vi "Main.vi"(11 "Module Admin":refnum<class "Delacor_lib_QMH_Cloneable Module Admin.lvclass">) -> ()   [LabVIEW 2024, in "Mensajes.lvlib"]
doc: "This template is based off of the Queued Message Handler design pattern and the Queued Message Handler project template that ships with LabVIEW.\n\nThe main difference is that the queue is private to this module and communication between modules is performed via Broadcast and Request events.\n\nRequest events are wrapped in public API methods and are handled in the Event Handling Loop (EHL) of this VI. Any module can register for Broadcast events sent by this module. The EHL generates messages based on user interface actions.\n\nThe Message Handling Loop (MHL) processes messages generated by the EHL, or by other messages. The messages are string values, so new messages can be added easily to the Message Cases case structure in the MHL. Each message cluster can also provide an optional value for Message Data, which is a variant that can be converted to whatever message-specific data is required.\n_____\nBased on DQMH Dev Tools: Project Template 7.1.0.1503."
uses:
  Mensajes.lvlib
  <vilib>/Delacor/Delacor QMH/Libraries/Cloneable Module Admin_class/Delacor_lib_QMH_Cloneable Module Admin.lvclass/Delacor_lib_QMH_Cloneable Module Admin.ctl
  <vilib>/Delacor/Delacor QMH/Libraries/Message Queue_class/Delacor_lib_QMH_Message Queue.lvclass/Delacor_lib_QMH_Message Queue.ctl
  <vilib>/Delacor/Delacor QMH/Libraries/Module Admin_class/Delacor_lib_QMH_Module Admin.lvclass/Delacor_lib_QMH_Module Admin.ctl
  <vilib>/Delacor/Delacor QMH/Libraries/Message Queue_class/Delacor_lib_QMH_Message Queue.lvclass
  Module Data--cluster.ctl
  <vilib>/Delacor/Delacor QMH/Libraries/Message Queue_class/Delacor_lib_QMH_Enqueue Message (Single).vi
  Stop Argument--cluster.ctl
  <vilib>/Delacor/Delacor QMH/Libraries/Cloneable Module Admin_class/Delacor_lib_QMH_Cloneable Module Admin.lvclass
  Draw FP in Subpanel Argument--cluster.ctl
  Remove From Subpanel Argument--cluster.ctl
  Despliega Mensaje Argument--cluster.ctl
  <vilib>/Utility/miscctls.llb/LVFontTypeDef.ctl
  Set Text Font Settings Argument--cluster.ctl
panel:
  out "Msg":string
  out "error out":errorcluster
  out "Status":string
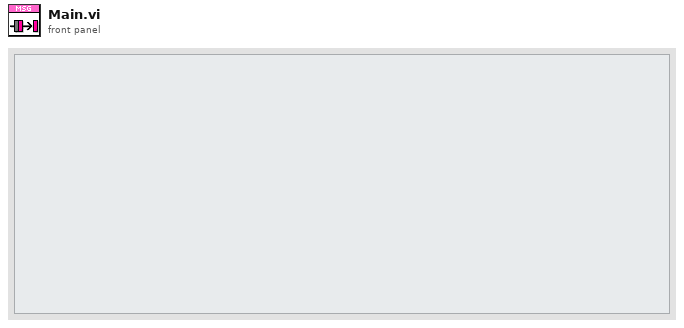
[diagram p1: front panel]
types:
  T1 = typedef "Mensajes.lvlib/Request Events--cluster.ctl" = cluster{"Stop Module":refnum<user-event>, "Show Panel":refnum<user-event>, "Hide Panel":refnum<user-event>, "Show Diagram":refnum<user-event>, "Get Module Execution Status":refnum<user-event>, "Draw FP in Subpanel":refnum<user-event>, "Remove From Subpanel":refnum<user-event>, "Despliega Mensaje":refnum<user-event>, "Set Text Font Settings":refnum<user-event>}
  T2 = typedef "Mensajes.lvlib/Module Data--cluster.ctl" = cluster{"Status":string, "Sub Panel":refnum<vi>, "Msg Ref":refnum<vi>}
  T3 = enum32{"invalid lock state", "Not Locked", "Locked (No Password)", "Password-protected"}
  T4 = typedef "Mensajes.lvlib/Stop Argument--cluster.ctl" = cluster{"Module ID":i32, "Origin":string, "Exit via Stop Module Req?":bool, "Wait for Module to stop?":bool}
  T5 = typedef "Mensajes.lvlib/Draw FP in Subpanel Argument--cluster.ctl" = cluster{"Module ID":i32, "Sub Panel":refnum<vi>}
  T6 = typedef "Mensajes.lvlib/Remove From Subpanel Argument--cluster.ctl" = cluster{"Module ID":i32, "Boolean":bool}
  T7 = typedef "Mensajes.lvlib/Despliega Mensaje Argument--cluster.ctl" = cluster{"Module ID":i32, "Mensaje":string}
  T8 = typedef "Mensajes.lvlib/Set Text Font Settings Argument--cluster.ctl" = cluster{"Module ID":i32, "Text.Font":T9}
  T9 = typedef "LVFontTypeDef.ctl" = cluster{"Font Name":string, "Size":u16, "Bold":bool, "Italic":bool, "Underline":bool, "Strikeout":bool, "Color":u32}
  T10 = enum32{"Invalid", "Standard", "Closed", "Hidden", "Minimized", "Maximized"}
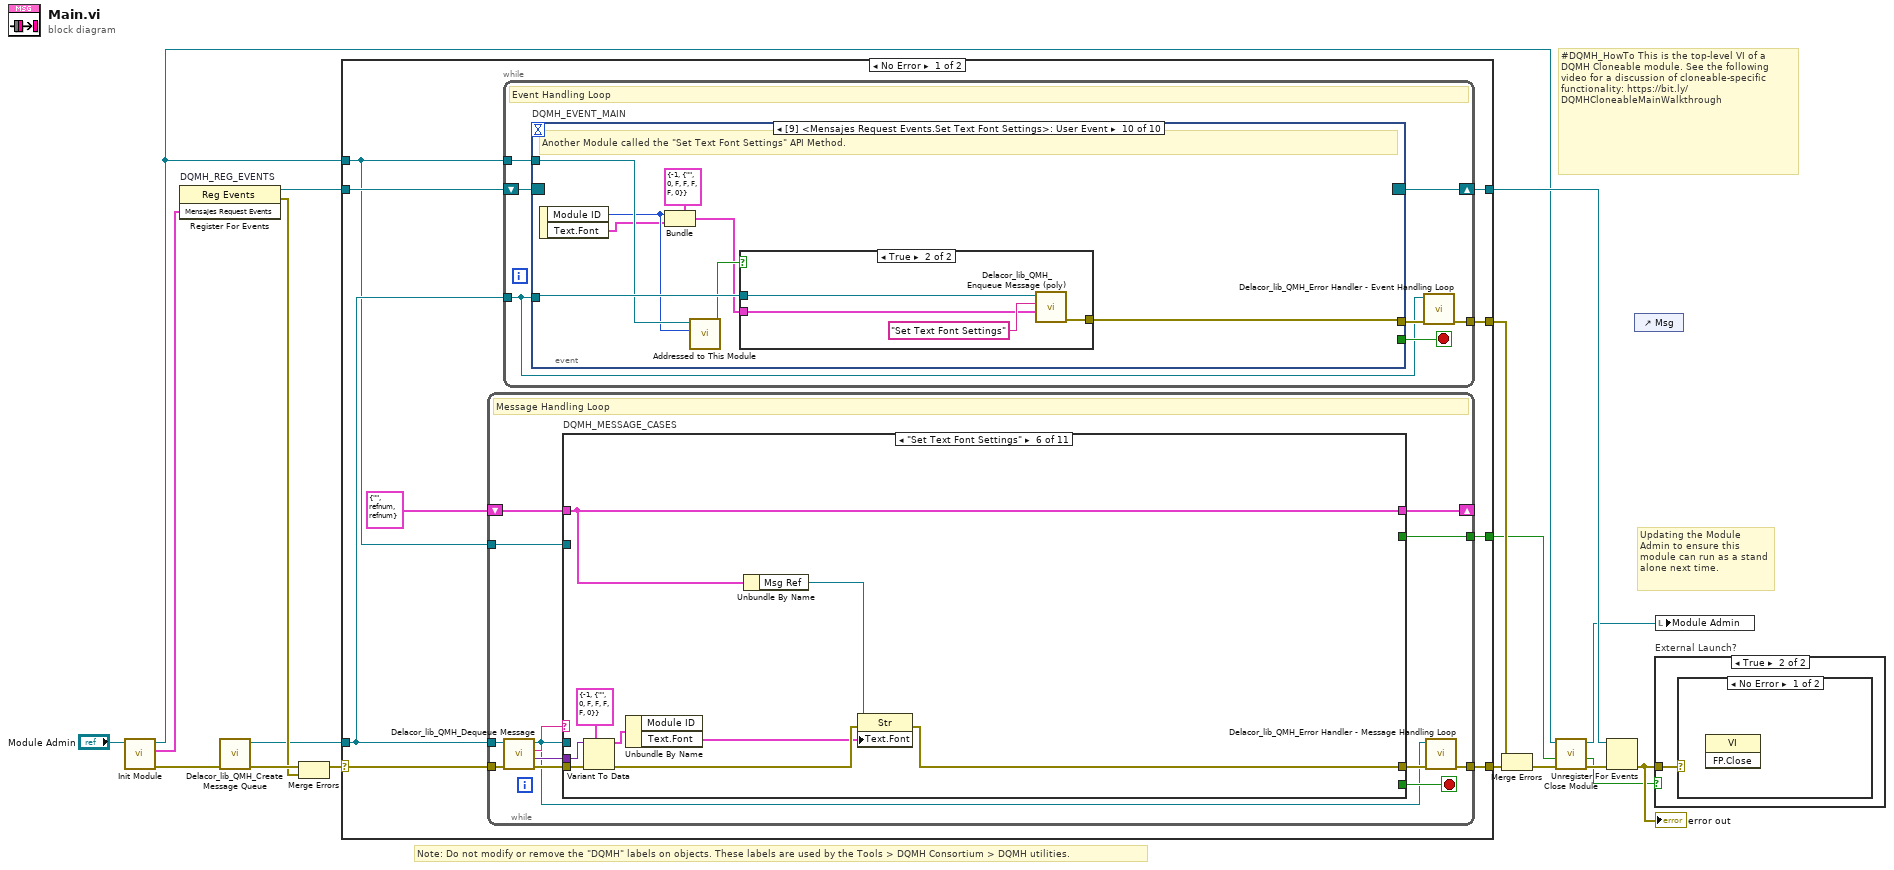
[diagram p0: block diagram]
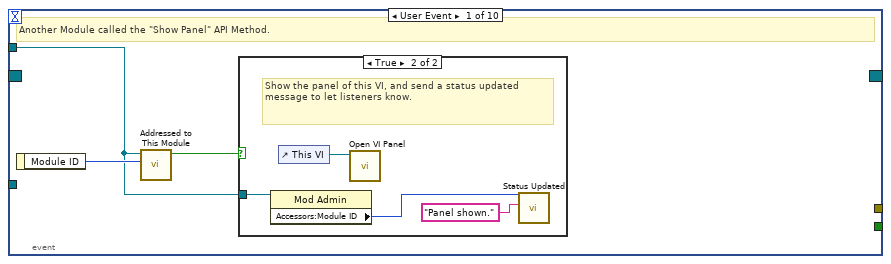
[diagram p2: hidden frame]
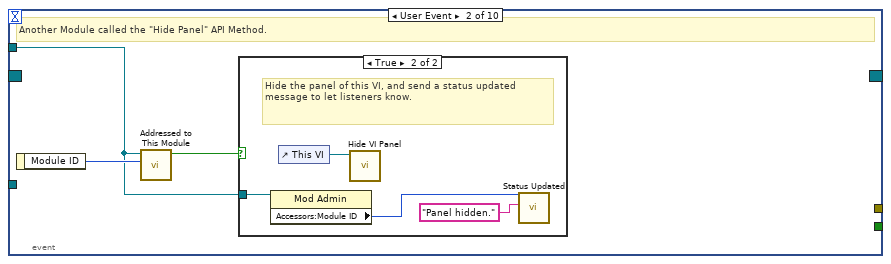
[diagram p4: hidden frame]
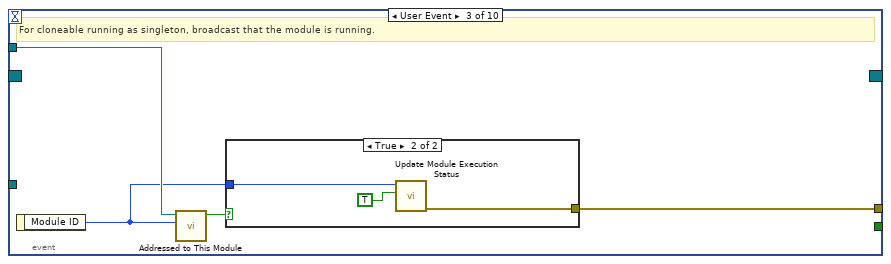
[diagram p6: hidden frame]
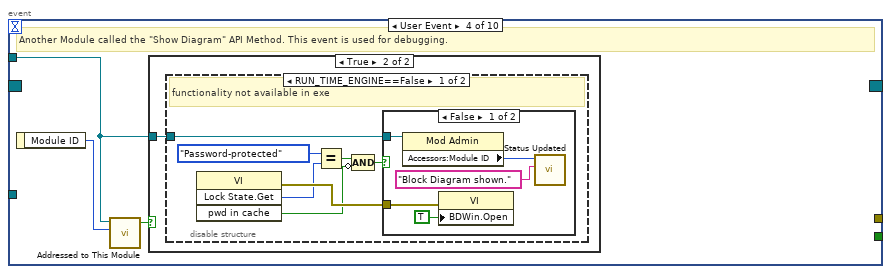
[diagram p8: hidden frame]
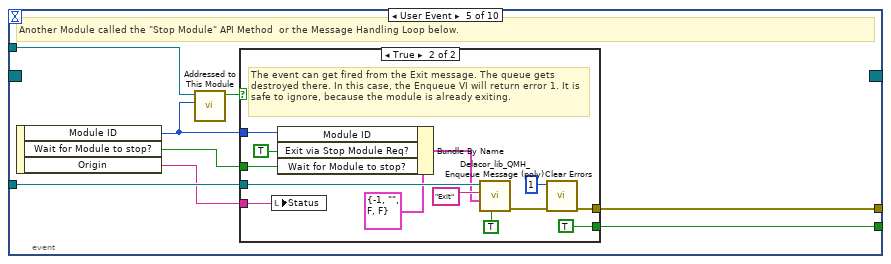
[diagram p12: hidden frame]
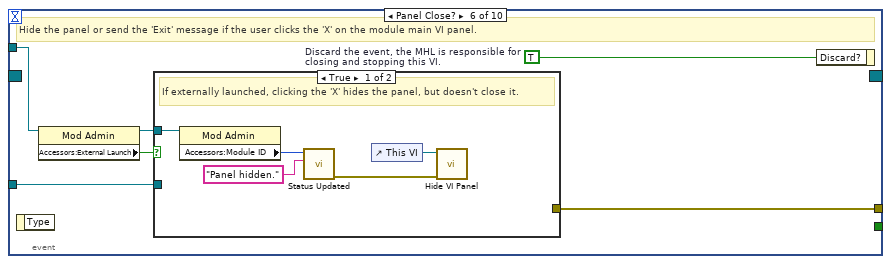
[diagram p14: hidden frame]
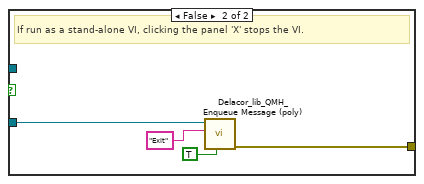
[diagram p15: hidden frame]
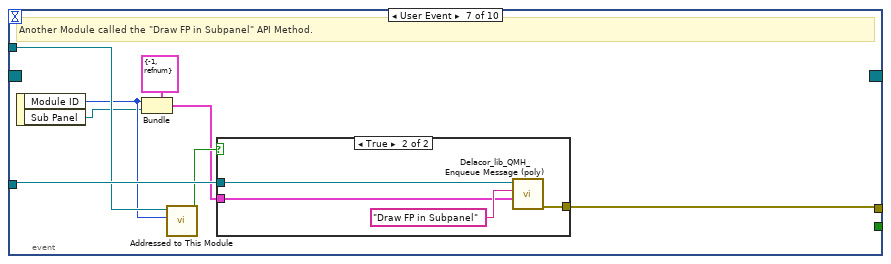
[diagram p16: hidden frame]
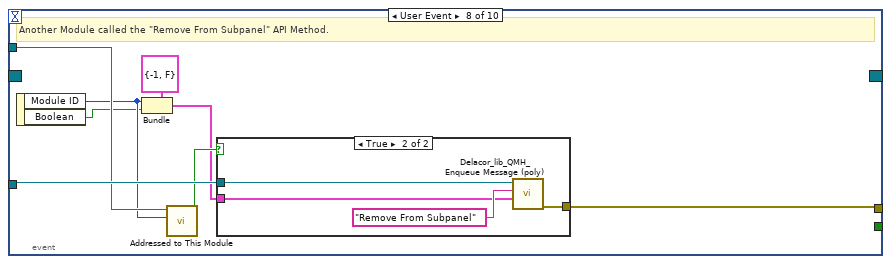
[diagram p18: hidden frame]
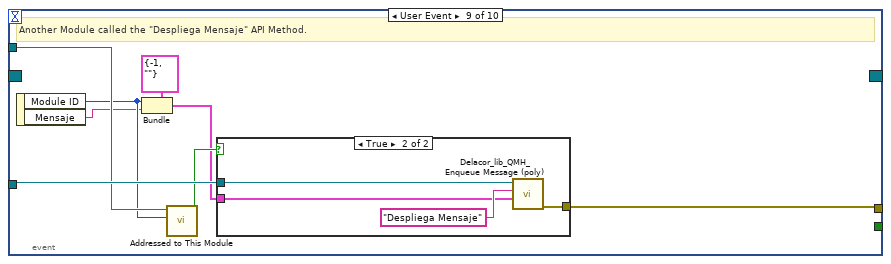
[diagram p20: hidden frame]
diagram:
  # "#DQMH_HowTo This is the top-level VI of a DQMH Cloneable module. See the following video for a discussion of cloneable-specific functionality: https://bit.ly/DQMHCloneableMainWalkthrough"
  # "Note: Do not modify or remove the \"DQMH\" labels on objects. These labels are used by the Tools > DQMH Consortium > DQMH utilities."
  # "Updating the Module Admin to ensure this module can run as a stand alone next time."
  n1 = call "Init Module.vi"("Cloneable Module Admin in"="Module Admin") -> ("error out"=w15:errorcluster, "Mensajes Request Events"=w7:T1, "Cloneable Module Admin out"=w4:refnum<class "Delacor_lib_QMH_Cloneable Module Admin.lvclass">)  [unwired: 8 in]
  n2 = register-events "DQMH_REG_EVENTS"(w7) -> (reference out=w8:refnum<event-registration>, error out=w10:errorcluster)  [unwired: 2 in]
  n3 = call <vilib>:"Delacor_lib_QMH_Create Message Queue.vi"("error in"=w15) -> ("error out"=w12:errorcluster, "Message Queue"=w6:refnum<class "Delacor_lib_QMH_Message Queue.lvclass">)  [unwired: 9 in]
  n4 = Merge Errors(w12, w10) -> (w11:errorcluster)
  n5 = case shown="No Error" w11 {
    selector: w11 -> [w25 w317]
    tunnel: [w27 w316] -> w16
    tunnel: [w24 w315] -> w9
    tunnel: w8 -> [w22 w315]
    tunnel: w6 -> [w21 w308]
    tunnel: [w26 _] -> w17
    tunnel: w4 -> [w20 w311]
    tunnel: [w19 _] -> w2
    frame No Error {
      n6 = while {
        tunnel: w21 -> [w156]
        shift-right: [w163] -> _
        shift-left: T2 {"Status"="", "Sub Panel"=refnum, "Msg Ref"=refnum} ("Data Cluster") -> [w164]
        tunnel: w25 -> [w167]
        tunnel: [w165] -> w27
        tunnel: w20 -> [w158]
        tunnel: [w157] -> w19
        stop <- w162 stop-if-true
        # "Message Handling Loop"
        n7 = call-dynamic "Delacor_lib_QMH_Dequeue Message.vi"("error in"=w167, "Message Queue in"=w156) -> ("error out"=w166:errorcluster, "Message Data"=w160:variant, "Message"=w161:string, "Message Queue out"=w159:refnum<class "Delacor_lib_QMH_Message Queue.lvclass">)  [unwired: 6 in]
        n8 = case "DQMH_MESSAGE_CASES" shown="\"Set Text Font Settings\"" w161 {
          selector: w161 -> [_ _ _ _ _ _ _ _ _ _ w297]
          tunnel: w159 -> [_ _ _ _ _ _ _ _ w261 w289 _]
          tunnel: w166 -> [w187 w191 w210 w230 w245 w254 w257 w259 w271 w295 w306]
          tunnel: [w185 w191 w206 w228 w243 w249 w256 w259 w267 w290 w307] -> w168
          tunnel: w164 -> [w178 w190 w196 w222 w244 w247 w255 w258 w265 w279 w304]
          tunnel: [w177 w190 w197 w218 w244 w247 w255 w258 w265 w279 w304] -> w163
          tunnel: [_ _ _ _ _ _ _ _ _ w288 _] -> w162
          tunnel: w160 -> [_ _ w205 w227 w242 w253 _ _ w264 w286 _]
          tunnel: w158 -> [w173 _ w194 w221 w238 _ _ _ w263 w281 w303]
          tunnel: [_ _ _ _ _ _ _ _ _ w284 _] -> w157
          frame "Initialize" {
            w171 = "Initial Message" ("Initial Message")
            # "#DQMH_CodeNeeded - Initialize the appearance of the front panel."
            # "Initialize - Any operation that needs to be done before the module can receive messages. Synchronize Caller Events.vi will inform Start Module.vi that the module has launched and is ready to receive messages. Module Did Init.vi will broadcast that the module initialized."
            n9 = call "Synchronize Caller Events.vi"("error in"=w187, "Module Admin"=w173) -> ("error out"=w186:errorcluster, "Module Admin out"=w172:refnum<class "Delacor_lib_QMH_Cloneable Module Admin.lvclass">)  [unwired: 8 in]
            n10 = property on="Property Node" class="Mod Admin"(reference=w172) -> ("Accessors:Module ID"=w170:i32, "Accessors:External Launch"=w174:bool)  [unwired: 1 in, 2 out]
            n11 = call "Module Name--constant.vi"("Module ID"=w170) -> ("Module Name"=w182:string)  [unwired: 10 in]
            n12 = property on="Property Node" class="VI"("Front Panel.Title"=w182) -> (reference out=w184:refnum<vi>, error out=w189:errorcluster)  [unwired: 2 in]
            n13 = Select(t=T10."Hidden" ("State"), s=w174, f=T10."Standard" ("State")) -> (s? t:f=w179:T10)
            n14 = control-ref of="Msg"() -> (w169:refnum<vi>)
            n15 = invoke on="Invoke Node" class="VI" method="FP.Open"(reference=w184, error in=w189, "State"=w179) -> (reference out=w183:refnum<vi>, error out=w188:errorcluster)  [unwired: 2 in, 3 out]
            n16 = Bundle By Name(cluster=w178, "Msg Ref"=w169, "Status"=w171) -> (w177:T2)
            n17 = invoke on="Invoke Node" class="VI" method="FP.Center"(reference=w183, error in=w188) -> ()  [unwired: 1 in, 3 out]
            n18 = call "Module Name--constant.vi"("Module ID"=w170) -> ("Module Name"=w175:string)  [unwired: 10 in]
            n19 = call "Module Did Init.vi"("error in"=w186, "Initialized?"=TRUE, "Origin"=w175, "Module ID"=w170) -> ("error out"=w185:errorcluster)  [unwired: 7 in]
            "Status" <- w171
          }
          frame "---Module Specific---" {
            # "Separator -- The following cases handle messages specific to this Module."
          }
          frame "Draw FP in Subpanel" {
            # "Draw FP in Subpanel"
            n20 = Variant To Data(error in=w210, type=T5 {"Module ID"=-1, "Sub Panel"=refnum} ("Draw FP in Subpanel Argument"), Variant=w205) -> (data=w203:T5, error out=w207:errorcluster)
            n21 = property class="Mod Admin"(reference=w194) -> ("Accessors:Module ID"=w193:i32)  [unwired: 1 in, 2 out]
            n22 = Unbundle By Name(w203) -> ("Sub Panel"=w195:refnum<vi>)
            n23 = control-ref of="This VI"() -> (w200:refnum<vi>)
            n24 = property class="VI"(reference=w200, error in=w207) -> (reference out=w199:refnum<vi>, error out=w208:errorcluster, "FP.State"=w198:T10)
            n25 = case shown="\"Closed\"" w198 {
              tunnel: [w211 w214] -> w201
              tunnel: [w212 w216] -> w209
              tunnel: w208 -> [w212 w215]
              tunnel: w199 -> [w211 w213]
              frame "Closed" {
              }
              frame "Standard", Default {
                n26 = invoke class="VI" method="FP.Close"(reference=w213, error in=w215) -> (reference out=w214:refnum<vi>, error out=w216:errorcluster)  [unwired: 1 in, 1 out]
              }
            }
            n27 = invoke class="SubPnl" method="Insert VI"(reference=w195, error in=w209, "VI Ref"=w201) -> (reference out=w202:refnum<vi>, error out=w206:errorcluster)  [unwired: 1 in, 2 out]
            n28 = call "Status Updated.vi"("error in"=w206, "Status"="Front Panel Inserted in Subpanel", "Module ID"=w193) -> ()  [unwired: 8 in, 1 out]
            n29 = Bundle By Name(cluster=w196, "Sub Panel"=w202) -> (w197:T2)
          }
          frame "Remove From Subpanel" {
            # "Remove From Subpanel"
            n30 = Variant To Data(error in=w230, type=T6 {"Module ID"=-1, "Boolean"=FALSE} ("Remove From Subpanel Argument"), Variant=w227) -> (data=w225:T6, error out=w229:errorcluster)
            n31 = Unbundle By Name(w225) -> ()  [unwired: 2 out]
            n32 = property class="Mod Admin"(reference=w221) -> ("Accessors:Module ID"=w220:i32)  [unwired: 1 in, 2 out]
            n33 = Unbundle By Name(w222) -> ("Sub Panel"=w224:refnum<vi>)
            n34 = Not A Number/Path/Refnum?(number/path/refnum=w224) -> (NaN/Path/Refnum?=w223:bool)
            n35 = case shown="False" w223 {
              tunnel: w229 -> [w234 w236]
              tunnel: [w233 w236] -> w228
              tunnel: w224 -> [w232 _]
              tunnel: ["Panel Removed from Subpanel" "This module has not been inserted into the subpanel"] -> w219
              frame False {
                n36 = invoke class="SubPnl" method="Remove VI"(reference=w232, error in=w234) -> (error out=w233:errorcluster)  [unwired: 1 in, 2 out]
              }
              frame True {
              }
            }
            n37 = Bundle By Name(cluster=w222, "Sub Panel"=refnum<vi> refnum) -> (w218:T2)
            n38 = call "Status Updated.vi"("error in"=w228, "Status"=w219, "Module ID"=w220) -> ()  [unwired: 8 in, 1 out]
          }
          frame "Despliega Mensaje" {
            n39 = Variant To Data(error in=w245, type=T7 {"Module ID"=-1, "Mensaje"=""} ("Despliega Mensaje Argument"), Variant=w242) -> (data=w240:T7, error out=w243:errorcluster)
            n40 = property class="Mod Admin"(reference=w238) -> ("Accessors:Module ID"=w237:i32)  [unwired: 1 in, 2 out]
            n41 = Unbundle By Name(w240) -> ("Mensaje"=w239:string)  [unwired: 1 out]
            "Msg" <- w239
            n42 = call "Status Updated.vi"("Status"=w239, "Module ID"=w237) -> ()  [unwired: 9 in, 1 out]
          }
          frame "Set Text Font Settings" {
            n43 = Variant To Data(error in=w254, type=T8 {"Module ID"=-1, "Text.Font"={"Font Name"="", "Size"=0, "Bold"=FALSE, "Italic"=FALSE, "Underline"=FALSE, "Strikeout"=FALSE, "Color"=0}} ("Set Text Font Settings Argument"), Variant=w253) -> (data=w251:T8, error out=w250:errorcluster)
            n44 = Unbundle By Name(w251) -> ("Text.Font"=w248:T9)  [unwired: 1 out]
            n45 = Unbundle By Name(w247) -> ("Msg Ref"=w246:refnum<vi>)
            n46 = property class="Str"(reference=w246, error in=w250, "Text.Font"=w248) -> (error out=w249:errorcluster)  [unwired: 1 out]
          }
          frame "---Copy This Frame---" {
            # "Duplicate this frame when creating new messages.  Change this comment in the duplicated frame to describe this message."
            n47 = Merge Errors(w257) -> (w256:errorcluster)
          }
          frame "---Exit and Error Handling---" {
            # "Separator - the following cases handle errors and exit messages."
          }
          frame "Error" {
            # "#DQMH_CodeRecommended - If the module is running in standalone mode (External Launch = FALSE), this code will pop up an error dialog and call the 'Exit' message if an error occurs. Add more fine-grained error management here."
            # "Error - Check the error message data and respond accordingly. This message is sent by the \"Error Handler\" VIs at the end of each loop in this application."
            n48 = property on="Property Node" class="Mod Admin"(reference=w263) -> ("Accessors:External Launch"=w262:bool, "Accessors:Module ID"=w260:i32)  [unwired: 1 in, 2 out]
            n49 = Variant To Data(error in=w271, type=errorcluster {"status"=FALSE, "code"=0, "source"=""} ("error constant"), Variant=w264) -> (data=w266:errorcluster, error out=w269:errorcluster)
            n50 = local write "error out"(w266) -> ()
            n51 = call "Error Reported.vi"("Error"=w266, "Module ID"=w260) -> ()  [unwired: 9 in, 1 out]
            n52 = case shown="False" w262 {
              tunnel: [w276 _] -> w268
              tunnel: w261 -> [w274 _]
              tunnel: w266 -> [w275 _]
              frame False {
                n53 = disable-structure shown="Default" {
                  disable-tunnel: w275 -> [w277 _]
                  frame condition #0 (active) {
                    # "If the module is running standalone, then pop up an error dialog and call the \"Exit\" message."
                    n54 = call <vilib>:"Simple Error Handler.vi"("error in (no error)"=w277) -> ()  [unwired: 4 in, 5 out]
                  }
                  frame condition #1 {
                    # "To prevent the Simple Error Handler VI from being loaded (e.g. when deploying to a Real-Time target), add the Conditional Disable Symbol \"DQMH_Disable_SEH\" to your project and set it to TRUE."
                  }
                }
                n55 = call-poly <vilib>:"Delacor_lib_QMH_Enqueue Message (poly).vi"("Priority Message? (F)"=TRUE, "Message"="Exit", "Message Queue in"=w274) -> ("error out"=w276:errorcluster)  [unwired: 7 in, 1 out]
              }
              frame True {
                # "If the module was launched externally, calling the Error Reported broadcast VI is the only action performed by the \"Error\" message. The module's caller can then process the error appropriately."
              }
            }
            n56 = Merge Errors(w269, w268) -> (w267:errorcluster)
          }
          frame "Exit" {
            w287 = 91  # 91: not all Exit messages will have an argument
            w288 = TRUE  # Stop the VI
            # "Release the message queue reference"
            # "#DQMH_CodeNeeded - Add any required cleanup code here."
            # "Exit - Exit the application."
            n57 = Variant To Data(error in=w295, type=T4 {"Module ID"=-1, "Origin"="", "Exit via Stop Module Req?"=FALSE, "Wait for Module to stop?"=FALSE} ("Stop Argument"), Variant=w286) -> (data=w283:T4, error out=w291:errorcluster)
            n58 = call <vilib>:"Clear Errors.vi"("error in (no error)"=w291, "specific error code to clear (0: all)"=w287) -> ("error out"=w294:errorcluster)  [unwired: 4 in, 1 out]
            n59 = property on="Property Node" class="Mod Admin"(reference=w281) -> ("Accessors:Module ID"=w280:i32)  [unwired: 1 in, 2 out]
            n60 = control-ref of="This VI"() -> (w282:refnum<vi>)
            n61 = call-dynamic "Delacor_lib_QMH_Release Message Queue.vi"("error in"=w294, "Message Queue"=w289) -> ("error out"=w293:errorcluster)  [unwired: 9 in]
            n62 = call "Handle Exit.vi"("Stop Argument"=w283, "Module Admin in"=w281, "VI reference"=w282) -> ("error out"=w292:errorcluster, "Wait for Stop?"=w284:bool)  [unwired: 7 in]
            n63 = Merge Errors(w293, w292) -> (w290:errorcluster)
            n64 = Unbundle By Name(w279) -> ("Sub Panel"=w278:refnum<vi>)
            n65 = call "Error Reported.vi"("Error"=w290, "Module ID"=w280) -> ()  [unwired: 9 in, 1 out]
            n66 = invoke class="SubPnl" method="Remove VI"(reference=w278) -> ()  [unwired: 2 in, 3 out]
          }
          frame Default {
            # "'Default' case only runs if there is a message that isn't defined in any of the other cases.  Output a programming error."
            n67 = property on="Property Node" class="Mod Admin"(reference=w303) -> ("Accessors:Module ID"=w302:i32)  [unwired: 1 in, 2 out]
            n68 = call "Module Name--constant.vi"("Module ID"=w302) -> ("Module Name"=w296:string)  [unwired: 10 in]
            n69 = Format Into String(format string="The invalid message string \"%s\" was received in the Message Handling Loop for module \"%s\".", w297, w296) -> (resulting string=w299:string)  [unwired: 2 in, 1 out]
            n70 = call <vilib>:"Error Cluster From Error Code.vi"("show call chain? (False)"=TRUE, "error message (\"\")"=w299, "error code (0)"=1) -> ("error out"=w305:errorcluster)  [unwired: 6 in]
            n71 = Merge Errors(w306, w305) -> (w307:errorcluster)
          }
        }
        n72 = call-dynamic "Delacor_lib_QMH_Error Handler - Message Handling Loop.vi"("error in"=w168, "Message Queue in"=w159) -> ("dup error in"=w165:errorcluster)  [unwired: 8 in, 1 out]
      }
      n73 = while {
        tunnel: w21 -> [w28]
        shift-right: [w31] -> w24
        shift-left: w22 -> [w32]
        tunnel: [w33] -> w26
        tunnel: w20 -> [w29]
        stop <- w30 stop-if-true
        # "Event Handling Loop"
        n74 = event "DQMH_EVENT_MAIN" shown="[9] <Mensajes Request Events.Set Text Font Settings>: User Event" {
          selector: w32 -> [_ _ _ _ _ _ _ _ _ _]
          dyn-events: [_ _ _ _ _ _ _ _ _ _] -> w31
          timeout: _ -> [_ _ _ _ _ _ _ _ _ _]
          tunnel: [_ _ _ _ w75 _ _ _ _ _] -> w30
          tunnel: w28 -> [_ _ _ _ w78 w95 w114 w126 w139 w151]
          tunnel: [_ _ w52 _ w79 w98 w115 w127 w132 w144] -> w34
          tunnel: w29 -> [w35 w42 w50 w56 w77 w96 w112 w124 w137 w149]
          event User Event {
            # "Another Module called the \"Show Panel\" API Method."
            n75 = event-data() -> ("Module ID"=w36:i32)  [unwired: 1 in]
            n76 = call "Addressed to This Module.vi"("Module ID from Argument"=w36, "Module Admin"=w35) -> ("Addressed to this instance?"=w37:bool)  [unwired: 8 in, 1 out]
            n77 = case shown="True" w37 {
              tunnel: w35 -> [_ w39]
              frame False {
              }
              frame True {
                # "Show the panel of this VI, and send a status updated message to let listeners know."
                n78 = property on="Property Node" class="Mod Admin"(reference=w39) -> ("Accessors:Module ID"=w38:i32)  [unwired: 1 in, 2 out]
                n79 = control-ref of="This VI"() -> (w41:refnum<vi>)
                n80 = call "Open VI Panel.vi"("VI"=w41) -> ()  [unwired: 10 in, 1 out]
                n81 = call "Status Updated.vi"("Status"="Panel shown." ("format string"), "Module ID"=w38) -> ()  [unwired: 9 in, 1 out]
              }
            }
          }
          event User Event {
            # "Another Module called the \"Hide Panel\" API Method."
            n82 = event-data() -> ("Module ID"=w43:i32)  [unwired: 1 in]
            n83 = call "Addressed to This Module.vi"("Module ID from Argument"=w43, "Module Admin"=w42) -> ("Addressed to this instance?"=w44:bool)  [unwired: 8 in, 1 out]
            n84 = case shown="True" w44 {
              tunnel: w42 -> [_ w46]
              frame False {
              }
              frame True {
                # "Hide the panel of this VI, and send a status updated message to let listeners know."
                n85 = property on="Property Node" class="Mod Admin"(reference=w46) -> ("Accessors:Module ID"=w45:i32)  [unwired: 1 in, 2 out]
                n86 = control-ref of="This VI"() -> (w48:refnum<vi>)
                n87 = call "Hide VI Panel.vi"("VI"=w48) -> ()  [unwired: 10 in, 1 out]
                n88 = call "Status Updated.vi"("Status"="Panel hidden." ("format string"), "Module ID"=w45) -> ()  [unwired: 9 in, 1 out]
              }
            }
          }
          event User Event {
            # "For cloneable running as singleton, broadcast that the module is running."
            n89 = event-data() -> ("Module ID"=w49:i32)  [unwired: 1 in]
            n90 = call "Addressed to This Module.vi"("Module ID from Argument"=w49, "Module Admin"=w50) -> ("Addressed to this instance?"=w51:bool)  [unwired: 8 in, 1 out]
            n91 = case shown="True" w51 {
              tunnel: [_ w55] -> w52
              tunnel: w49 -> [_ w54]
              frame False {
              }
              frame True {
                n92 = call "Update Module Execution Status.vi"("Running?"=TRUE, "Module ID"=w54) -> ("error out"=w55:errorcluster)  [unwired: 9 in]
              }
            }
          }
          event User Event {
            # "Another Module called the \"Show Diagram\" API Method. This event is used for debugging."
            n93 = event-data() -> ("Module ID"=w57:i32)  [unwired: 1 in]
            n94 = call "Addressed to This Module.vi"("Module ID from Argument"=w57, "Module Admin"=w56) -> ("Addressed to this instance?"=w58:bool)  [unwired: 8 in, 1 out]
            n95 = case shown="True" w58 {
              tunnel: w56 -> [_ w59]
              frame False {
              }
              frame True {
                n96 = disable-structure shown="RUN_TIME_ENGINE==False" {
                  disable-tunnel: w59 -> [w60 _]
                  frame condition #0 (active) {
                    # "functionality not available in exe"
                    n97 = invoke on="Invoke Node" class="VI" method="Lock State.Get"() -> (error out=w66:errorcluster, "Get Lock State"=w65:T3, "pwd in cache"=w62:bool)  [unwired: 4 in, 1 out]
                    n98 = Equal?(x=T3."Password-protected", y=w65) -> (x = y?=w63:bool)
                    n99 = Compound Arithmetic op=AND(w63, invert w62) -> (w61:bool)
                    n100 = case shown="False" w61 {
                      tunnel: w66 -> [w71 _]
                      tunnel: w60 -> [w68 _]
                      frame False {
                        n101 = property on="Property Node" class="Mod Admin"(reference=w68) -> ("Accessors:Module ID"=w67:i32)  [unwired: 1 in, 2 out]
                        n102 = property on="Property Node" class="VI"(error in=w71, "BDWin.Open"=TRUE ("Block Diagram Window:Open")) -> ()  [unwired: 1 in, 2 out]
                        n103 = call "Status Updated.vi"("Status"="Block Diagram shown." ("format string"), "Module ID"=w67) -> ()  [unwired: 9 in, 1 out]
                      }
                      frame True {
                        # "Password-protected VI, and the password is not in the cache. Do not show the diagram."
                      }
                    }
                  }
                  frame condition #1 {
                  }
                }
              }
            }
          }
          event User Event {
            # "Another Module called the \"Stop Module\" API Method  or the Message Handling Loop below."
            n104 = event-data() -> ("Module ID"=w73:i32, "Wait for Module to stop?"=w74:bool, "Origin"=w72:string)  [unwired: 1 in]
            n105 = call "Addressed to This Module.vi"("Module ID from Argument"=w73, "Module Admin"=w77) -> ("Addressed to this instance?"=w76:bool)  [unwired: 8 in, 1 out]
            n106 = case shown="True" w76 {
              tunnel: [_ w91] -> w79
              tunnel: w78 -> [_ w87]
              tunnel: [_ TRUE] -> w75
              tunnel: w74 -> [_ w82]
              tunnel: w73 -> [_ w84]
              tunnel: w72 -> [_ w80]
              frame False {
              }
              frame True {
                # "The event can get fired from the Exit message. The queue gets destroyed there. In this case, the Enqueue VI will return error 1. It is safe to ignore, because the module is already exiting."
                n107 = local write "Status"(w80) -> ()
                n108 = Bundle By Name(cluster=T4 {"Module ID"=-1, "Origin"="", "Exit via Stop Module Req?"=FALSE, "Wait for Module to stop?"=FALSE} ("Stop Argument"), "Module ID"=w84, "Exit via Stop Module Req?"=TRUE, "Wait for Module to stop?"=w82) -> (w81:T4)
                n109 = call-poly <vilib>:"Delacor_lib_QMH_Enqueue Message (poly).vi"("Priority Message? (F)"=TRUE, "Message Data"=w81, "Message"="Exit", "Message Queue in"=w87) -> ("error out"=w92:errorcluster)  [unwired: 6 in, 1 out]
                n110 = call <vilib>:"Clear Errors.vi"("error in (no error)"=w92, "specific error code to clear (0: all)"=1) -> ("error out"=w91:errorcluster)  [unwired: 4 in, 1 out]
              }
            }
          }
          event Panel Close? {
            w97 = TRUE  # Discard the event, the MHL is responsible for closing and stopping this VI.
            # "Hide the panel or send the 'Exit' message if the user clicks the 'X' on the module main VI panel."
            n111 = event-data() -> ()  [unwired: 1 in, 1 out]
            n112 = property on="Property Node" class="Mod Admin"(reference=w96) -> (reference out=w93:refnum<class "Delacor_lib_QMH_Cloneable Module Admin.lvclass">, "Accessors:External Launch"=w94:bool)  [unwired: 1 in, 1 out]
            n113 = case shown="True" w94 {
              tunnel: w95 -> [_ w106]
              tunnel: [_ w107] -> w98
              tunnel: w93 -> [w100 _]
              frame True {
                # "If externally launched, clicking the 'X' hides the panel, but doesn't close it."
                n114 = property on="Property Node" class="Mod Admin"(reference=w100) -> ("Accessors:Module ID"=w99:i32)  [unwired: 1 in, 2 out]
                n115 = call "Status Updated.vi"("Status"="Panel hidden." ("format string"), "Module ID"=w99) -> ("error out"=w103:errorcluster)  [unwired: 9 in]
                n116 = control-ref of="This VI"() -> (w102:refnum<vi>)
                n117 = call "Hide VI Panel.vi"("error in"=w103, "VI"=w102) -> ()  [unwired: 9 in, 1 out]
              }
              frame False {
                # "If run as a stand-alone VI, clicking the panel 'X' stops the VI."
                n118 = call-poly <vilib>:"Delacor_lib_QMH_Enqueue Message (poly).vi"("Priority Message? (F)"=TRUE, "Message"="Exit", "Message Queue in"=w106) -> ("error out"=w107:errorcluster)  [unwired: 7 in, 1 out]
              }
            }
            n119 = event-data ("Event Filter Node")("Discard?"=w97) -> ()  [unwired: 1 in, 1 out]
          }
          event User Event {
            # "Another Module called the \"Draw FP in Subpanel\" API Method."
            n120 = event-data() -> ("Module ID"=w109:i32, "Sub Panel"=w108:refnum<vi>)  [unwired: 1 in]
            n121 = Bundle(cluster=T5 {"Module ID"=-1, "Sub Panel"=refnum} ("Draw FP in Subpanel Argument"), "Module ID"=w109, "Sub Panel"=w108) -> (w110:T5)
            n122 = call "Addressed to This Module.vi"("Module ID from Argument"=w109, "Module Admin"=w112) -> ("Addressed to this instance?"=w113:bool)  [unwired: 8 in, 1 out]
            n123 = case shown="True" w113 {
              tunnel: w114 -> [_ w118]
              tunnel: w110 -> [_ w116]
              tunnel: [_ w119] -> w115
              frame False {
              }
              frame True {
                n124 = call-poly <vilib>:"Delacor_lib_QMH_Enqueue Message (poly).vi"("Message Data"=w116, "Message"="Draw FP in Subpanel", "Message Queue in"=w118) -> ("error out"=w119:errorcluster)  [unwired: 7 in, 1 out]
              }
            }
          }
          event User Event {
            # "Another Module called the \"Remove From Subpanel\" API Method."
            n125 = event-data() -> ("Module ID"=w121:i32, "Boolean"=w120:bool)  [unwired: 1 in]
            n126 = Bundle(cluster=T6 {"Module ID"=-1, "Boolean"=FALSE} ("Remove From Subpanel Argument"), "Module ID"=w121, "Boolean"=w120) -> (w122:T6)
            n127 = call "Addressed to This Module.vi"("Module ID from Argument"=w121, "Module Admin"=w124) -> ("Addressed to this instance?"=w125:bool)  [unwired: 8 in, 1 out]
            n128 = case shown="True" w125 {
              tunnel: w126 -> [_ w130]
              tunnel: w122 -> [_ w128]
              tunnel: [_ w131] -> w127
              frame False {
              }
              frame True {
                n129 = call-poly <vilib>:"Delacor_lib_QMH_Enqueue Message (poly).vi"("Message Data"=w128, "Message"="Remove From Subpanel", "Message Queue in"=w130) -> ("error out"=w131:errorcluster)  [unwired: 7 in, 1 out]
              }
            }
          }
          event User Event {
            # "Another Module called the \"Despliega Mensaje\" API Method."
            n130 = event-data() -> ("Module ID"=w134:i32, "Mensaje"=w133:string)  [unwired: 1 in]
            n131 = Bundle(cluster=T7 {"Module ID"=-1, "Mensaje"=""} ("Despliega Mensaje Argument"), "Module ID"=w134, "Mensaje"=w133) -> (w135:T7)
            n132 = call "Addressed to This Module.vi"("Module ID from Argument"=w134, "Module Admin"=w137) -> ("Addressed to this instance?"=w138:bool)  [unwired: 8 in, 1 out]
            n133 = case shown="True" w138 {
              tunnel: w139 -> [_ w143]
              tunnel: w135 -> [_ w141]
              tunnel: [_ w140] -> w132
              frame False {
              }
              frame True {
                n134 = call-poly <vilib>:"Delacor_lib_QMH_Enqueue Message (poly).vi"("Message Data"=w141, "Message"="Despliega Mensaje", "Message Queue in"=w143) -> ("error out"=w140:errorcluster)  [unwired: 7 in, 1 out]
              }
            }
          }
          event User Event {
            # "Another Module called the \"Set Text Font Settings\" API Method."
            n135 = event-data() -> ("Module ID"=w146:i32, "Text.Font"=w145:T9)  [unwired: 1 in]
            n136 = Bundle(cluster=T8 {"Module ID"=-1, "Text.Font"={"Font Name"="", "Size"=0, "Bold"=FALSE, "Italic"=FALSE, "Underline"=FALSE, "Strikeout"=FALSE, "Color"=0}} ("Set Text Font Settings Argument"), "Module ID"=w146, "Text.Font"=w145) -> (w147:T8)
            n137 = call "Addressed to This Module.vi"("Module ID from Argument"=w146, "Module Admin"=w149) -> ("Addressed to this instance?"=w150:bool)  [unwired: 8 in, 1 out]
            n138 = case shown="True" w150 {
              tunnel: w151 -> [_ w155]
              tunnel: w147 -> [_ w153]
              tunnel: [_ w152] -> w144
              frame False {
              }
              frame True {
                n139 = call-poly <vilib>:"Delacor_lib_QMH_Enqueue Message (poly).vi"("Message Data"=w153, "Message"="Set Text Font Settings", "Message Queue in"=w155) -> ("error out"=w152:errorcluster)  [unwired: 7 in, 1 out]
              }
            }
          }
        }
        n140 = call-dynamic "Delacor_lib_QMH_Error Handler - Event Handling Loop.vi"("error in"=w34, "Message Queue in"=w28) -> ("dup error in"=w33:errorcluster)  [unwired: 8 in, 1 out]
      }
    }
    frame Error {
      n141 = call "Synchronize Caller Events.vi"("Module Admin"=w311) -> ("Module Admin out"=w310:refnum<class "Delacor_lib_QMH_Cloneable Module Admin.lvclass">)  [unwired: 9 in, 1 out]
      n142 = property on="Property Node" class="Mod Admin"(reference=w310) -> ("Accessors:Module ID"=w309:i32)  [unwired: 1 in, 2 out]
      n143 = call-dynamic "Delacor_lib_QMH_Release Message Queue.vi"("error in"=w317, "Message Queue"=w308) -> ("error out"=w316:errorcluster)  [unwired: 9 in]
      n144 = call "Module Name--constant.vi"("Module ID"=w309) -> ("Module Name"=w314:string)  [unwired: 10 in]
      n145 = Format Into String(format string="An error occurred during initialization. %s is no longer running.", w314) -> (resulting string=w312:string)  [unwired: 2 in, 1 out]
      n146 = call "Error Reported.vi"("Additional Information"=w312, "Error"=w316, "Module ID"=w309) -> ()  [unwired: 8 in, 1 out]
    }
  }
  n147 = Merge Errors(w17, w16) -> (w18:errorcluster)
  n148 = call "Close Module.vi"("error in"=w18, "Wait for stop?"=w2, "Module Admin in"=w4) -> ("error out"=w14:errorcluster, "External Launch"=w1:bool, "Module Admin out"=w3:refnum<class "Delacor_lib_QMH_Cloneable Module Admin.lvclass">)  [unwired: 6 in]
  n149 = Unregister For Events(event registration refnum=w9, error in=w14) -> (error out=w13:errorcluster)
  "error out" <- w13
  n150 = control-ref of="Msg"() -> ()  [unwired: 1 out]
  n151 = case "External Launch?" shown="True" w1 {
    tunnel: w13 -> [_ w318]
    frame False {
    }
    frame True {
      n152 = case shown="No Error" w318 {
        frame No Error {
          n153 = invoke class="VI" method="FP.Close"() -> ()  [unwired: 3 in, 3 out]
        }
        frame Error {
          n154 = disable-structure shown="Default" {
            frame condition #0 (active) {
              n155 = invoke class="VI" method="FP.Open"("Activate"=TRUE ("Activate?")) -> ()  [unwired: 4 in, 5 out]
            }
            frame condition #1 {
              # "Don't show panel on error if running inside a built EXE."
            }
          }
        }
      }
    }
  }
  n156 = local write "Module Admin"(w3) -> ()
